vi "CAN_example.vi"() -> ()   [LabVIEW 2012]
uses:
  <vilib>/nican/nicantsk.llb/CAN Interface.ctl
  <vilib>/nican/nicantsk.llb/CAN Mode.ctl
  <vilib>/nican/nicantsk.llb/CAN Read Multi Chan Single Samp 1D Dbl.vi
  <vilib>/nican/nicantsk.llb/CAN Write Multi Chan Single Samp 1D Dbl.vi
panel:
  in  "stop 2":bool
  out "byte0":dbl
  out "byte1":dbl
  in  "Interface":T1 items=["CAN0"=0, "CAN1"=1, "CAN2"=2, "CAN3"=3, "CAN4"=4, "CAN5"=5, "CAN6"=6, "CAN7"=7, "CAN8"=8, "CAN9"=9, "CAN10"=10, "CAN11"=11, "CAN12"=12, "CAN13"=13, "CAN14"=14, "CAN15"=15, "CAN16"=16, "CAN17"=17, "CAN18"=18, "CAN19"=19, "CAN20"=20, "CAN21"=21, "CAN22"=22, "CAN23"=23, "CAN24"=24, "CAN25"=25, "CAN26"=26, "CAN27"=27, "CAN28"=28, "CAN29"=29, "CAN30"=30, "CAN31"=31, "CAN32"=32, "CAN33"=33, "CAN34"=34, "CAN35"=35, "CAN36"=36, "CAN37"=37, "CAN38"=38, "CAN39"=39, "CAN40"=40, "CAN41"=41, "CAN42"=42, "CAN43"=43, "CAN44"=44, "CAN45"=45, "CAN46"=46, "CAN47"=47, "CAN48"=48, "CAN49"=49, "CAN50"=50, "CAN51"=51, "CAN52"=52, "CAN53"=53, "CAN54"=54, "CAN55"=55, "CAN56"=56, "CAN57"=57, "CAN58"=58, "CAN59"=59, "CAN60"=60, "CAN61"=61, "CAN62"=62, "CAN63"=63, "MAX default"=64, "CAN256 (Virtual)"=256, "CAN257 (Virtual)"=257]
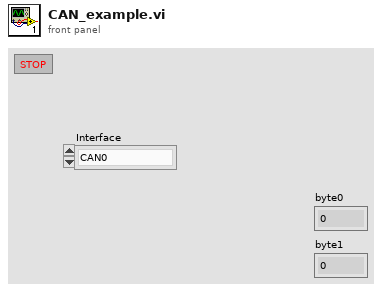
[diagram p1: front panel]
types:
  T1 = typedef "CAN Interface.ctl" = u16
  T2 = typedef "CAN Mode.ctl" = u16
  T3 = typedef "CAN Task Reference.ctl" = u32
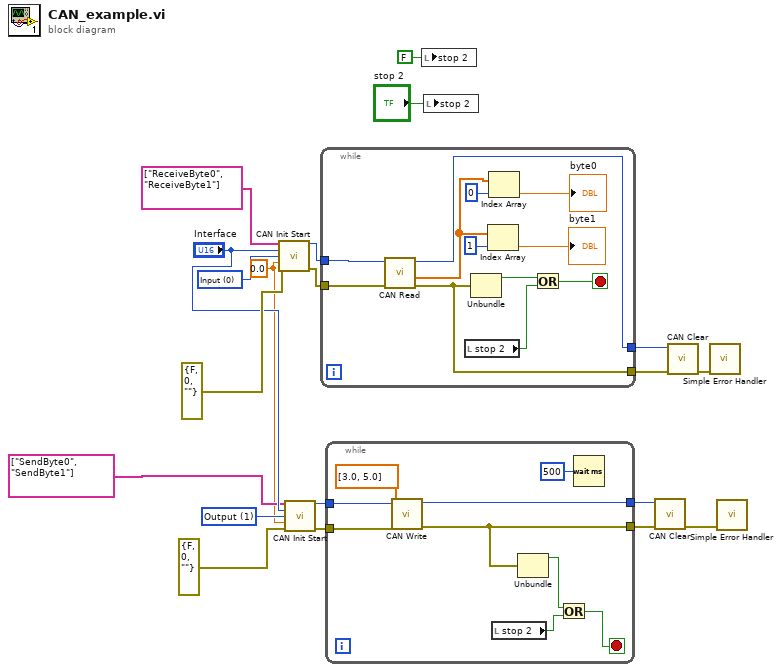
[diagram p0: block diagram]
diagram:
  w3 = 0.0 ("sample rate")
  w12 = T2 1 items=["Input", "Output", "Timestamped Input", "Output Recent"] ("mode")
  w20 = T2 0 items=["Input", "Output", "Timestamped Input", "Output Recent"] ("mode")
  n1 = call <vilib>:"CAN Init Start.vi"("channel list"=string[] ["ReceiveByte0", "ReceiveByte1"] ("Channel List"), "interface"="Interface", "mode"=w20, "sample rate"=w3, "error in (no error)"=errorcluster {"status"=FALSE, "code"=0, "source"=""}) -> ("task reference out"=w19:T3, "error out"=w18:errorcluster)  [unwired: 9 in]
  n2 = call <vilib>:"CAN Init Start.vi"("channel list"=string[] ["SendByte0", "SendByte1"] ("Channel List 2"), "interface"="Interface", "mode"=w12, "sample rate"=w3, "error in (no error)"=errorcluster {"status"=FALSE, "code"=0, "source"=""}) -> ("task reference out"=w10:T3, "error out"=w9:errorcluster)  [unwired: 9 in]
  n3 = while {
    tunnel: w19 -> [w32]
    tunnel: w18 -> [w31]
    tunnel: [w25] -> w16
    tunnel: [w30] -> w15
    stop <- w28 stop-if-true
    n4 = call-poly <vilib>:"CAN Read.vi"("error in (no error)"=w31, "task reference in"=w32) -> ("error out"=w30:errorcluster, "multi-chan single-samp 1D dbl"=w22:dbl[], "task reference out"=w25:T3)  [unwired: 6 in, 1 out]
    n5 = local read "stop 2"() -> (w21:bool)
    n6 = Unbundle(w30) -> ("status"=w29:bool)  [unwired: 2 out]
    n7 = Index Array(array=w22, index=1) -> (element=→"byte1":dbl)
    n8 = Index Array(array=w22, index=0) -> (element=→"byte0":dbl)
    n9 = Or(x=w29, y=w21) -> (x .or. y?=w28:bool)
  }
  n10 = while {
    tunnel: w10 -> [w41]
    tunnel: w9 -> [w40]
    tunnel: [w39] -> w8
    tunnel: [w38] -> w7
    stop <- w36 stop-if-true
    n11 = call-poly <vilib>:"CAN Write.vi"("error in (no error)"=w40, "multi-chan single-samp 1D dbl"=dbl[] [3.0, 5.0], "task reference in"=w41) -> ("error out"=w38:errorcluster, "task reference out"=w39:T3)  [unwired: 7 in]
    n12 = local read "stop 2"() -> (w33:bool)
    n13 = Unbundle(w38) -> ("status"=w37:bool)  [unwired: 2 out]
    n14 = Or(x=w37, y=w33) -> (x .or. y?=w36:bool)
    n15 = Wait (ms)(milliseconds to wait=u32 500) -> ()  [unwired: 1 out]
  }
  n16 = local write "stop 2"(FALSE ("stop 2")) -> ()
  n17 = local write "stop 2"("stop 2") -> ()
  n18 = call <vilib>:"CAN Clear.vi"("error in (no error)"=w7, "task reference in"=w8) -> ("error out"=w6:errorcluster)  [unwired: 9 in]
  n19 = call <vilib>:"CAN Clear.vi"("error in (no error)"=w15, "task reference in"=w16) -> ("error out"=w14:errorcluster)  [unwired: 9 in]
  n20 = call <vilib>:"Simple Error Handler.vi"("error in (no error)"=w14) -> ()  [unwired: 4 in, 5 out]
  n21 = call <vilib>:"Simple Error Handler.vi"("error in (no error)"=w6) -> ()  [unwired: 4 in, 5 out]
